vi "XBMC JSON Type To Enum.vi"() -> ()   [LabVIEW 2013, in "LMH-Kodi.lvlib"]
uses:
  LMH-Kodi.lvlib
  <vilib>/MakerHub/Toolbox/Private/Scripting/LMH-Scripting.lvlib
panel:
  in  "Name Override":string="Input.Action"
  out "Error Out":errorcluster
  in  "Enum Dest Dir":path=path "C:/Program Files (x86)/National Instruments/LabVIEW 2013/vi.lib/LabVIEW Hacker/XBMC/Private/Type Defs"
  in  "JSON Array":string="\"enums\": [\n\t\t\t\t\"left\",\n\t\t\t\t\"right\",\n\t\t\t\t\"up\",\n\t\t\t\t\"down\",\n\t\t\t\t\"pageup\",\n\t\t\t\t\"pagedown\",\n\t\t\t\t\"select\",\n\t\t\t\t\"highlight\",\n\t\t\t\t\"parentdir\",\n\t\t\t\t\"parentfolder\",\n\t\t\t\t\"back\",\n\t\t\t\t\"previousmenu\",\n\t\t\t\t\"info\",\n\t\t\t\t\"pause\",\n\t\t\t\t\"stop\",\n\t\t\t\t\"skipnext\",\n\t\t\t\t\"skipprevious\",\n\t\t\t\t\"fullscreen\",\n\t\t\t\t\"aspectratio\",\n\t\t\t\t\"stepforward\",\n\t\t\t\t\"stepback\",\n\t\t\t\t\"bigstepforward\",\n\t\t\t\t\"bigstepback\",\n\t\t\t\t\"chapterorbigstepforward\",\n\t\t\t\t\"chapterorbigstepback\",\n\t\t\t\t\"osd\",\n\t\t\t\t\"showsubtitles\",\n\t\t\t\t\"nextsubtitle\",\n\t\t\t\t\"codecinfo\",\n\t\t\t\t\"nextpicture\",\n\t\t\t\t\"previouspicture\",\n\t\t\t\t\"zoomout\",\n\t\t\t\t\"zoomin\",\n\t\t\t\t\"playlist\",\n\t\t\t\t\"queue\",\n\t\t\t\t\"zoomnormal\",\n\t\t\t\t\"zoomlevel1\",\n\t\t\t\t\"zoomlevel2\",\n\t\t\t\t\"zoomlevel3\",\n\t\t\t\t\"zoomlevel4\",\n\t\t\t\t\"zoomlevel5\",\n\t\t\t\t\"zoomlevel6\",\n\t\t\t\t\"zoomlevel7\",\n\t\t\t\t\"zoomlevel8\",\n\t\t\t\t\"zoomlevel9\",\n\t\t\t\t\"nextcalibration\",\n\t\t\t\t\"resetcalibration\",\n\t\t\t\t\"analogmove\",\n\t\t\t\t\"rotate\",\n\t\t\t\t\"rotateccw\",\n\t\t\t\t\"close\",\n\t\t\t\t\"subtitledelayminus\",\n\t\t\t\t\"subtitledelay\",\n\t\t\t\t\"subtitledelayplus\",\n\t\t\t\t\"audiodelayminus\",\n\t\t\t\t\"audiodelay\",\n\t\t\t\t\"audiodelayplus\",\n\t\t\t\t\"subtitleshiftup\",\n\t\t\t\t\"subtitleshiftdown\",\n\t\t\t\t\"subtitlealign\",\n\t\t\t\t\"audionextlanguage\",\n\t\t\t\t\"verticalshiftup\",\n\t\t\t\t\"verticalshiftdown\",\n\t\t\t\t\"nextresolution\",\n\t\t\t\t\"audiotoggledigital\",\n\t\t\t\t\"number0\",\n\t\t\t\t\"number1\",\n\t\t\t\t\"number2\",\n\t\t\t\t\"number3\",\n\t\t\t\t\"number4\",\n\t\t\t\t\"number5\",\n\t\t\t\t\"number6\",\n\t\t\t\t\"number7\",\n\t\t\t\t\"number8\",\n\t\t\t\t\"number9\",\n\t\t\t\t\"osdleft\",\n\t\t\t\t\"osdright\",\n\t\t\t\t\"osdup\",\n\t\t\t\t\"osddown\",\n\t\t\t\t\"osdselect\",\n\t\t\t\t\"osdvalueplus\",\n\t\t\t\t\"osdvalueminus\",\n\t\t\t\t\"smallstepback\",\n\t\t\t\t\"fastforward\",\n\t\t\t\t\"rewind\",\n\t\t\t\t\"play\",\n\t\t\t\t\"playpause\",\n\t\t\t\t\"switchplayer\",\n\t\t\t\t\"delete\",\n\t\t\t\t\"copy\",\n\t\t\t\t\"move\",\n\t\t\t\t\"mplayerosd\",\n\t\t\t\t\"hidesubmenu\",\n\t\t\t\t\"screenshot\",\n\t\t\t\t\"rename\",\n\t\t\t\t\"togglewatched\",\n\t\t\t\t\"scanitem\",\n\t\t\t\t\"reloadkeymaps\",\n\t\t\t\t\"volumeup\",\n\t\t\t\t\"volumedown\",\n\t\t\t\t\"mute\",\n\t\t\t\t\"backspace\",\n\t\t\t\t\"scrollup\",\n\t\t\t\t\"scrolldown\",\n\t\t\t\t\"analogfastforward\",\n\t\t\t\t\"analogrewind\",\n\t\t\t\t\"moveitemup\",\n\t\t\t\t\"moveitemdown\",\n\t\t\t\t\"contextmenu\",\n\t\t\t\t\"shift\",\n\t\t\t\t\"symbols\",\n\t\t\t\t\"cursorleft\",\n\t\t\t\t\"cursorright\",\n\t\t\t\t\"showtime\",\n\t\t\t\t\"analogseekforward\",\n\t\t\t\t\"analogseekback\",\n\t\t\t\t\"showpreset\",\n\t\t\t\t\"presetlist\",\n\t\t\t\t\"nextpreset\",\n\t\t\t\t\"previouspreset\",\n\t\t\t\t\"lockpreset\",\n\t\t\t\t\"randompreset\",\n\t\t\t\t\"increasevisrating\",\n\t\t\t\t\"decreasevisrating\",\n\t\t\t\t\"showvideomenu\",\n\t\t\t\t\"enter\",\n\t\t\t\t\"increaserating\",\n\t\t\t\t\"decreaserating\",\n\t\t\t\t\"togglefullscreen\",\n\t\t\t\t\"nextscene\",\n\t\t\t\t\"previousscene\",\n\t\t\t\t\"nextletter\",\n\t\t\t\t\"prevletter\",\n\t\t\t\t\"jumpsms2\",\n\t\t\t\t\"jumpsms3\",\n\t\t\t\t\"jumpsms4\",\n\t\t\t\t\"jumpsms5\",\n\t\t\t\t\"jumpsms6\",\n\t\t\t\t\"jumpsms7\",\n\t\t\t\t\"jumpsms8\",\n\t\t\t\t\"jumpsms9\",\n\t\t\t\t\"filter\",\n\t\t\t\t\"filterclear\",\n\t\t\t\t\"filtersms2\",\n\t\t\t\t\"filtersms3\",\n\t\t\t\t\"filtersms4\",\n\t\t\t\t\"filtersms5\",\n\t\t\t\t\"filtersms6\",\n\t\t\t\t\"filtersms7\",\n\t\t\t\t\"filtersms8\",\n\t\t\t\t\"filtersms9\",\n\t\t\t\t\"firstpage\",\n\t\t\t\t\"lastpage\",\n\t\t\t\t\"guiprofile\",\n\t\t\t\t\"red\",\n\t\t\t\t\"green\",\n\t\t\t\t\"yellow\",\n\t\t\t\t\"blue\",\n\t\t\t\t\"increasepar\",\n\t\t\t\t\"decreasepar\",\n\t\t\t\t\"volampup\",\n\t\t\t\t\"volampdown\",\n\t\t\t\t\"createbookmark\",\n\t\t\t\t\"createepisodebookmark\",\n\t\t\t\t\"settingsreset\",\n\t\t\t\t\"settingslevelchange\",\n\t\t\t\t\"stereomode\",\n\t\t\t\t\"nextstereomode\",\n\t\t\t\t\"previousstereomode\",\n\t\t\t\t\"togglestereomode\",\n\t\t\t\t\"stereomodetomono\",\n\t\t\t\t\"channelup\",\n\t\t\t\t\"channeldown\",\n\t\t\t\t\"previouschannelgroup\",\n\t\t\t\t\"nextchannelgroup\",\n\t\t\t\t\"playpvr\",\n\t\t\t\t\"playpvrtv\",\n\t\t\t\t\"playpvrradio\",\n\t\t\t\t\"record\",\n\t\t\t\t\"leftclick\",\n\t\t\t\t\"rightclick\",\n\t\t\t\t\"middleclick\",\n\t\t\t\t\"doubleclick\",\n\t\t\t\t\"wheelup\",\n\t\t\t\t\"wheeldown\",\n\t\t\t\t\"mousedrag\",\n\t\t\t\t\"mousemove\",\n\t\t\t\t\"tap\",\n\t\t\t\t\"longpress\",\n\t\t\t\t\"pangesture\",\n\t\t\t\t\"zoomgesture\",\n\t\t\t\t\"rotategesture\",\n\t\t\t\t\"swipeleft\",\n\t\t\t\t\"swiperight\",\n\t\t\t\t\"swipeup\",\n\t\t\t\t\"swipedown\",\n\t\t\t\t\"noop\"\n\t\t\t]"
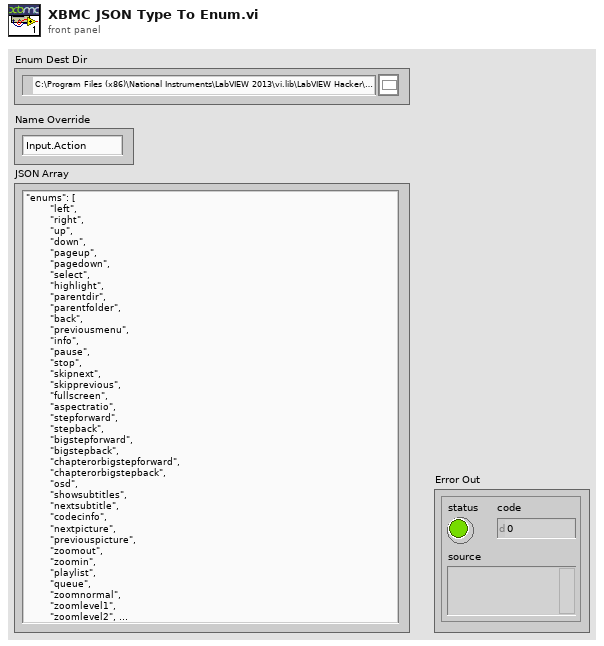
[diagram p1: front panel]
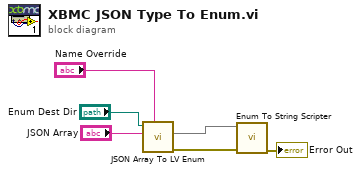
[diagram p0: block diagram]
diagram:
  n1 = call <vilib>:"JSON Array To LV Enum.vi"("Name Override"="Name Override", "JSON Array"="JSON Array", "Enum Dest Dir"="Enum Dest Dir") -> ("Error Out"=w3:errorcluster, 2:w2)  [unwired: 7 in]
  n2 = call <vilib>:"Enum To String Scripter.vi"("Error In"=w3, "Enum Path"=w2) -> ("Error Out"=→"Error Out":errorcluster)  [unwired: 9 in]
